vi "simple sine gen.vi"(7 "Source":T1={"source"=TRUE, "source type"=FALSE, "Amplitude"=1.0, "Period (steps)"=100.0} {"Amplitude" scale=0.0..1.0; "Period (steps)" scale=1.0..1000.0}) -> (8 "output":dbl)   [LabVIEW 2019]
doc: "This subvi is a one-shot kernal of sine or square wave generation using an unitialized shift register."
uses:
  typedefs/periodic signal control.ctl
panel:
  out "call counter":dbl
  # "Single Shot Sine Generator Kernel"
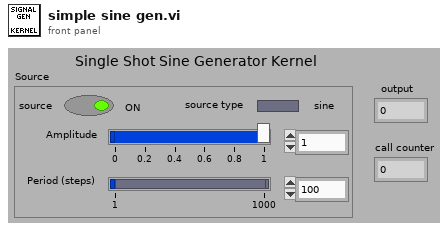
[diagram p1: front panel]
types:
  T1 = typedef "periodic signal control.ctl" = cluster{"source":bool, "source type":bool, "Amplitude":dbl, "Period (steps)":dbl}
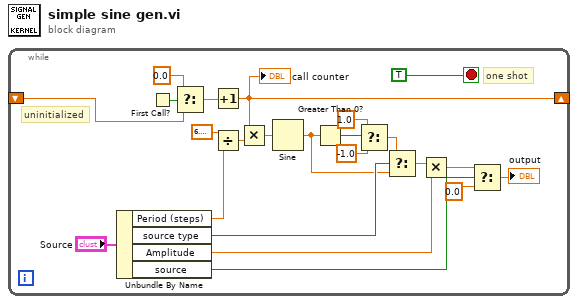
[diagram p0: block diagram]
diagram:
  n1 = while {
    shift-right: [w15] -> _
    shift-left: _ -> [w20]
    stop <- TRUE stop-if-true
    # "uninitialized"
    # "one shot"
    n2 = Unbundle By Name("Source") -> ("Period (steps)"=w13:dbl, "source type"=w6:bool, "Amplitude"=w5:dbl, "source"=w3:bool)
    n3 = First Call?() -> (First Call?: T/F=w21:bool)
    n4 = Select(t=0.0, s=w21, f=w20) -> (s? t:f=w22:dbl)
    n5 = Increment(x=w22) -> (x+1=w15:dbl)
    "call counter" <- w15
    n6 = Divide(x=6.283185307179586, y=w13) -> (x/y=w16:dbl)
    n7 = Multiply(x=w15, y=w16) -> (x*y=w17:dbl)
    n8 = Sine(x=w17) -> (sin(x)=w2:dbl)
    n9 = Greater Than 0?(x=w2) -> (x > 0?=w9:bool)
    n10 = Select(t=1.0, s=w9, f=-1.0) -> (s? t:f=w1:dbl)
    n11 = Select(t=w1, s=w6, f=w2) -> (s? t:f=w4:dbl)
    n12 = Multiply(x=w4, y=w5) -> (x*y=w12:dbl)
    n13 = Select(t=w12, s=w3, f=0.0) -> (s? t:f=→"output":dbl)
  }
